vi "DataStream_RT_Main Send Loop.vi"() -> ()   [LabVIEW 2020]
uses:
  Utility/Global_STOP.vi
panel:
  in  "Timeout":i32=1000
  out "cyle time":dbl
  out "Remote Endpoint Destroyed":bool
  out "Is Writable?":bool
  out "Is Connected":bool
  out "Error":errorcluster
  out "timed out?":bool
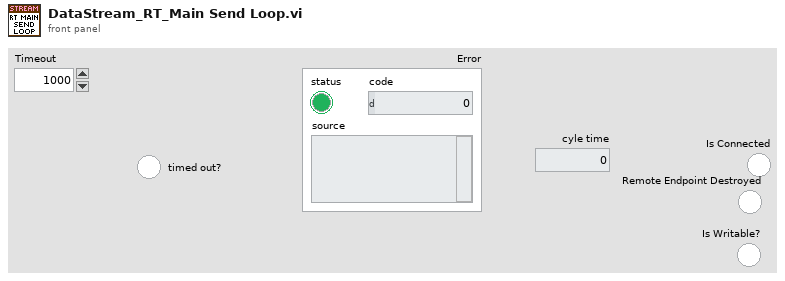
[diagram p1: front panel]
types:
  T1 = typedef "Cluster_DataStream_RT Writer Refs.ctl" = cluster{"Writer Data Ref":refnum<k21>}
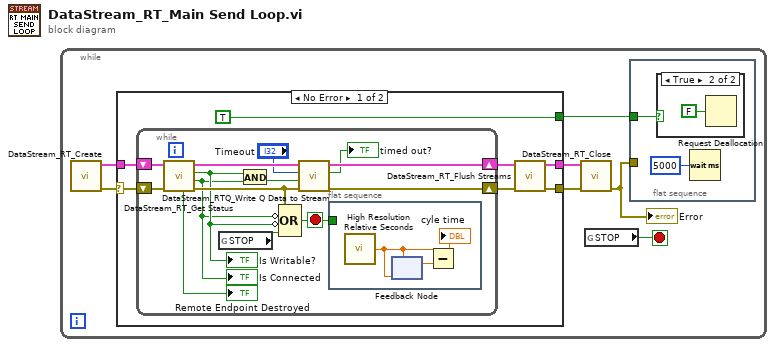
[diagram p0: block diagram]
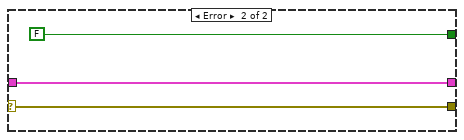
[diagram p3: hidden frame]
diagram:
  n1 = while {
    stop <- w7 stop-if-true
    n2 = call "DataStream_RT_Create.vi"() -> ("Error Out"=w4:errorcluster, "Stream Writer Ref Out"=w5:T1)  [unwired: 10 in]
    n3 = case shown="No Error" w4 {
      selector: w4 -> [w11 w37]
      tunnel: [w15 w37] -> w2
      tunnel: w5 -> [w17 w35]
      tunnel: [TRUE FALSE] -> w6
      tunnel: [w12 w35] -> w3
      frame No Error {
        n4 = while {
          shift-right: [w30] -> w13
          shift-left: w17 -> [w28]
          shift-right: [w24] -> w16
          shift-left: w11 -> [w29]
          stop <- w23 stop-if-true
          n5 = call "DataStream_RT_Get Status.vi"("Error"=w29, "Stream Writer Ref"=w28) -> ("Error Out"=w25:errorcluster, "Writable Out"=w19:bool, "Connected Out"=w20:bool, "Stream Writer Ref Out"=w27:T1, "RemoteEndptDestroyed Out"=→"Remote Endpoint Destroyed":bool)  [unwired: 5 in]
          "Is Connected" <- w19
          "Is Writable?" <- w20
          n6 = global read "Global_STOP.vi" "STOP"() -> (w31:bool)
          n7 = And(x=w20, y=w19) -> (x .and. y?=w18:bool)
          n8 = Compound Arithmetic op=OR(w25, invert w19, invert w20, w31) -> (w23:bool)
          n9 = call "DataStream_RTQ_Write Q Data to Stream.vi"("Error"=w25, "Connected"=w18, "Time"="Timeout", "Stream Writer Ref"=w27) -> ("Error Out"=w24:errorcluster, "Timed Out? Out"=→"timed out?":bool, "Stream Writer Ref Out"=w30:T1)  [unwired: 5 in]
          n10 = flat-sequence {
            tunnel: w23 -> [_]
            frame #0 {
              n11 = call <vilib>:"High Resolution Relative Seconds.vi"() -> ("relative seconds"=w33:dbl)
              n12 = feedback-in #1(w33) -> ()
              n13 = feedback #1(w33) -> (w34:dbl)
              n14 = Subtract(x=w33, y=w34) -> (x-y=→"cyle time":dbl)
            }
          }
        }
        n15 = call "DataStream_RT_Flush Streams.vi"("Error"=w16, "Stream Writer Ref"=w13) -> ("Error Out"=w15:errorcluster, "Stream Writer Ref Out"=w12:T1)  [unwired: 8 in]
      }
      frame Error {
      }
    }
    n16 = call "DataStream_RT_Close.vi"("Error"=w2, "Stream Ref"=w3) -> ("Error Out"=w1:errorcluster)  [unwired: 9 in]
    "Error" <- w1
    n17 = global read "Global_STOP.vi" "STOP"() -> (w7:bool)
    n18 = flat-sequence {
      tunnel: w6 -> [w8]
      tunnel: w1 -> [_]
      frame #0 {
        n19 = case shown="True" w8 {
          frame False {
          }
          frame True {
            n20 = Request Deallocation(FALSE ("flag")) -> ()
          }
        }
        n21 = Wait (ms)(milliseconds to wait=u32 5000) -> ()  [unwired: 1 out]
      }
    }
  }
